vi "M04 Smart Grid.vi"(11 "EV3 in":T1) -> (3 "EV3 out":T1)   [LabVIEW 2016]
uses:
  <vilib>/NXT/Subs/LVHSConnector.ctl
  <vilib>/NXT/LegoClasses/BrickReference/BrickReference.lvclass
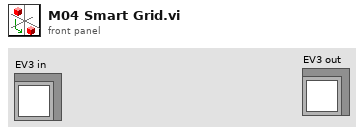
[diagram p1: front panel]
types:
  T1 = typedef "LVHSConnector.ctl" = refnum<class "BrickReference.lvclass">
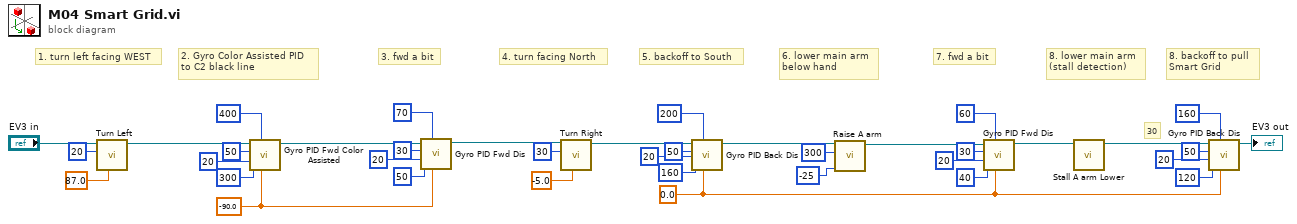
[diagram p0: block diagram]
diagram:
  w6 = sgl 0.0 ("Target angle")
  w25 = sgl -90.0 ("Target angle")
  # "30"
  # "7. fwd a bit"
  # "6. lower main arm\nbelow hand"
  # "8. backoff to pull\nSmart Grid"
  # "8. lower main arm\n(stall detection)"
  # "5. backoff to South"
  # "4. turn facing North"
  # "3. fwd a bit"
  # "2. Gyro Color Assisted PID\nto C2 black line"
  # "1. turn left facing WEST"
  n1 = call "Turn Left.vi"("Turning angle"=sgl 87.0, "Motor B (right)"=i8 20, "EV3 in"="EV3 in") -> ("EV3 out"=w35:T1)  [unwired: 8 in]
  n2 = call "Gyro PID Fwd Color Assisted.vi"("Target angle"=w25, "Threshold to Color"=400, "Threshold to slow"=300, "Min. speed"=20, "Max. speed"=50, "EV3 in"=w35) -> ("EV3 out"=w30:T1)  [unwired: 5 in]
  n3 = call "Gyro PID Fwd Dis.vi"("Target angle"=w25, "Threshold to stop"=70, "Threshold to slow"=50, "Min. speed"=20, "Max. speed"=30, "EV3 in"=w30) -> ("EV3 out"=w24:T1)  [unwired: 5 in]
  n4 = call "Turn Right.vi"("Turning angle"=sgl -5.0, "Motor B (right)"=i8 30, "EV3 in"=w24) -> ("EV3 out"=w21:T1)  [unwired: 8 in]
  n5 = call "Gyro PID Back Dis.vi"("Target angle"=w6, "Threshold to stop"=200, "Threshold to slow"=160, "Min. speed"=20, "Max. speed"=50, "EV3 in"=w21) -> ("EV3 out"=w4:T1)  [unwired: 5 in]
  n6 = call "Raise A arm.vi"("Power"=i8 -25 ("Speed 1"), "Rotation"=300, "EV3 in"=w4) -> ("EV3 out"=w1:T1)  [unwired: 8 in]
  n7 = call "Gyro PID Fwd Dis.vi"("Target angle"=w6, "Threshold to stop"=60, "Threshold to slow"=40, "Min. speed"=20, "Max. speed"=30, "EV3 in"=w1) -> ("EV3 out"=w11:T1)  [unwired: 5 in]
  n8 = call "Stall A arm Lower.vi"("NXT/EV3"=w11) -> ("NXT/EV3"=w16:T1)  [unwired: 10 in]
  n9 = call "Gyro PID Back Dis.vi"("Target angle"=w6, "Threshold to stop"=160, "Threshold to slow"=120, "Min. speed"=20, "Max. speed"=50, "EV3 in"=w16) -> ("EV3 out"=→"EV3 out":T1)  [unwired: 5 in]
